vi "Insert Channels and Preserve Value.vi"(7 "channel block":T1 {"buffer offset" format="%d bytes"}, 8 "error in (no error)":errorcluster, 9 "channels buffer index in":u64, 10 "channels buffer in":dbl[](array[numeric]), 11 "Buffer in":refnum<class "Memory Buffer.lvclass">) -> (0 "error out":errorcluster, 1 "channels buffer index out":u64, 2 "channels buffer out":dbl[](array[numeric]), 3 "Buffer out":refnum<class "Memory Buffer.lvclass">)   [LabVIEW 2017, in "Data Sharing Framework Engine.lvlib" / "Memory Buffer.lvclass"]
uses:
  Memory Buffer.lvclass
  Type Definitions/DSF Runtime Channel Block.ctl
  Configuration/1.0.0/Public/Controls/DSF Data Type.ctl
  Write 1D Array of U64.vi
  Write 1D Array of U32.vi
  Write 1D Array of U16.vi
  Write 1D Array of U8.vi
  Write 1D Array of I64.vi
  Write 1D Array of I32.vi
  Write 1D Array of I16.vi
  Write 1D Array of I8.vi
  Write 1D Array of Double.vi
  Write 1D Array of Single.vi
  Write 1D Array of Boolean.vi
  Data Sharing Framework Engine.lvlib
  Configuration/1.0.0/Data Sharing Framework Configuration.lvlib
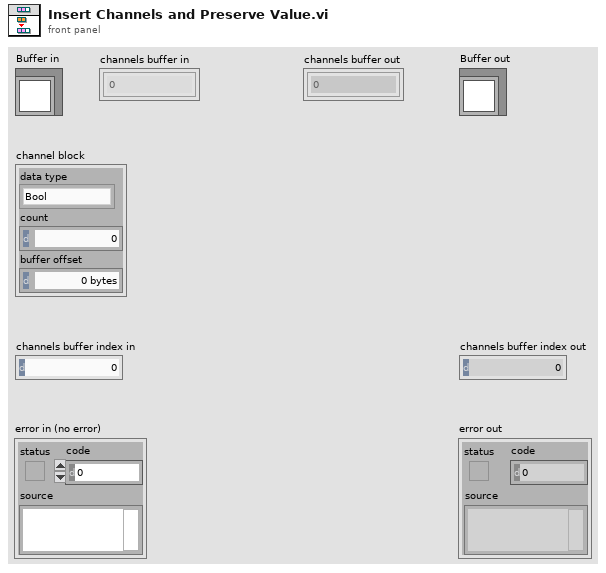
[diagram p1: front panel]
types:
  T1 = typedef "Data Sharing Framework Engine.lvlib/DSF Runtime Channel Block.ctl" = cluster{"data type":T2, "count":u64, "buffer offset":u64}
  T2 = typedef "Data Sharing Framework Configuration.lvlib/DSF Data Type.ctl" = enum8{"Bool", "SGL", "DBL", "I8", "I16", "I32", "I64", "U8", "U16", "U32", "U64"}
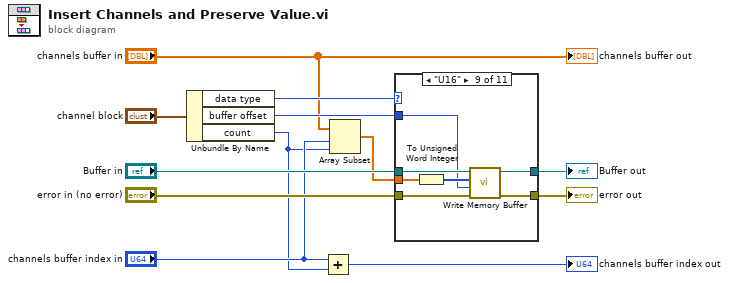
[diagram p0: block diagram]
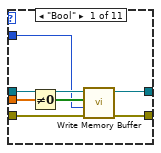
[diagram p2: hidden frame]
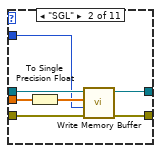
[diagram p3: hidden frame]
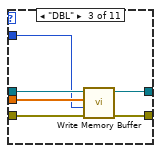
[diagram p4: hidden frame]
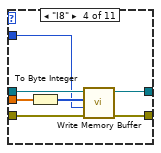
[diagram p5: hidden frame]
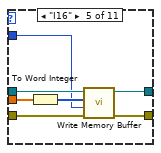
[diagram p6: hidden frame]
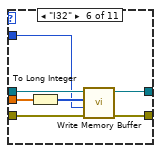
[diagram p7: hidden frame]
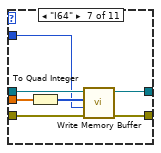
[diagram p8: hidden frame]
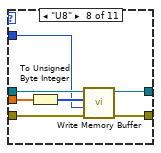
[diagram p9: hidden frame]
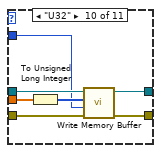
[diagram p10: hidden frame]
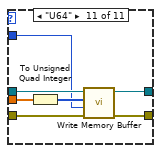
[diagram p11: hidden frame]
diagram:
  n1 = Unbundle By Name("channel block") -> ("data type"=w9:T2, "buffer offset"=w12:u64, "count"=w2:u64)
  n2 = Add(x="channels buffer index in", y=w2) -> (x+y=→"channels buffer index out":u64)
  n3 = Array Subset(array="channels buffer in", index="channels buffer index in", length=w2) -> (w6:dbl[])
  n4 = case shown="\"U16\"" w9 {
    tunnel: "Buffer in" -> [w19 w26 w32 w39 w46 w53 w60 w67 w74 w81 w88]
    tunnel: w6 -> [w14 w21 w28 w34 w41 w48 w55 w62 w69 w76 w83]
    tunnel: "error in (no error)" -> [w18 w25 w31 w38 w45 w52 w59 w66 w73 w80 w87]
    tunnel: [w17 w24 w30 w37 w44 w51 w58 w65 w72 w79 w86] -> w10
    tunnel: w12 -> [w15 w22 w27 w35 w42 w49 w56 w63 w70 w77 w84]
    tunnel: [w13 w20 w29 w33 w40 w47 w54 w61 w68 w75 w82] -> w7
    frame "Bool" {
      n5 = Not Equal To 0?(x=w14) -> (x != 0?=w16:bool[])
      n6 = call-poly "Write Memory Buffer.vi"("error in (no error)"=w18, "offset (0)"=w15, "buffer in"=w16, "Buffer in"=w19) -> ("error out"=w17:errorcluster, "Buffer out"=w13:refnum<class "Memory Buffer.lvclass">)  [unwired: 4 in, 2 out]
    }
    frame "SGL" {
      n7 = To Single Precision Float(number=w21) -> (single precision float=w23:sgl[])
      n8 = call-poly "Write Memory Buffer.vi"("error in (no error)"=w25, "offset (0)"=w22, "buffer in"=w23, "Buffer in"=w26) -> ("error out"=w24:errorcluster, "Buffer out"=w20:refnum<class "Memory Buffer.lvclass">)  [unwired: 4 in, 2 out]
    }
    frame "DBL" {
      n9 = call-poly "Write Memory Buffer.vi"("error in (no error)"=w31, "offset (0)"=w27, "buffer in"=w28, "Buffer in"=w32) -> ("error out"=w30:errorcluster, "Buffer out"=w29:refnum<class "Memory Buffer.lvclass">)  [unwired: 4 in, 2 out]
    }
    frame "I8" {
      n10 = To Byte Integer(number=w34) -> (8bit integer=w36:i8[])
      n11 = call-poly "Write Memory Buffer.vi"("error in (no error)"=w38, "offset (0)"=w35, "buffer in"=w36, "Buffer in"=w39) -> ("error out"=w37:errorcluster, "Buffer out"=w33:refnum<class "Memory Buffer.lvclass">)  [unwired: 4 in, 2 out]
    }
    frame "I16" {
      n12 = To Word Integer(number=w41) -> (16bit integer=w43:i16[])
      n13 = call-poly "Write Memory Buffer.vi"("error in (no error)"=w45, "offset (0)"=w42, "buffer in"=w43, "Buffer in"=w46) -> ("error out"=w44:errorcluster, "Buffer out"=w40:refnum<class "Memory Buffer.lvclass">)  [unwired: 4 in, 2 out]
    }
    frame "I32" {
      n14 = To Long Integer(number=w48) -> (32bit integer=w50:i32[])
      n15 = call-poly "Write Memory Buffer.vi"("error in (no error)"=w52, "offset (0)"=w49, "buffer in"=w50, "Buffer in"=w53) -> ("error out"=w51:errorcluster, "Buffer out"=w47:refnum<class "Memory Buffer.lvclass">)  [unwired: 4 in, 2 out]
    }
    frame "I64" {
      n16 = To Quad Integer(1:w55) -> (0:w57:i64[])
      n17 = call-poly "Write Memory Buffer.vi"("error in (no error)"=w59, "offset (0)"=w56, "buffer in"=w57, "Buffer in"=w60) -> ("error out"=w58:errorcluster, "Buffer out"=w54:refnum<class "Memory Buffer.lvclass">)  [unwired: 4 in, 2 out]
    }
    frame "U8" {
      n18 = To Unsigned Byte Integer(number=w62) -> (unsigned 8bit integer=w64:u8[])
      n19 = call-poly "Write Memory Buffer.vi"("error in (no error)"=w66, "offset (0)"=w63, "buffer in"=w64, "Buffer in"=w67) -> ("error out"=w65:errorcluster, "Buffer out"=w61:refnum<class "Memory Buffer.lvclass">)  [unwired: 4 in, 2 out]
    }
    frame "U16" {
      n20 = To Unsigned Word Integer(number=w69) -> (unsigned 16bit integer=w71:u16[])
      n21 = call-poly "Write Memory Buffer.vi"("error in (no error)"=w73, "offset (0)"=w70, "buffer in"=w71, "Buffer in"=w74) -> ("error out"=w72:errorcluster, "Buffer out"=w68:refnum<class "Memory Buffer.lvclass">)  [unwired: 4 in, 2 out]
    }
    frame "U32" {
      n22 = To Unsigned Long Integer(number=w76) -> (unsigned 32bit integer=w78:u32[])
      n23 = call-poly "Write Memory Buffer.vi"("error in (no error)"=w80, "offset (0)"=w77, "buffer in"=w78, "Buffer in"=w81) -> ("error out"=w79:errorcluster, "Buffer out"=w75:refnum<class "Memory Buffer.lvclass">)  [unwired: 4 in, 2 out]
    }
    frame "U64" {
      n24 = To Unsigned Quad Integer(1:w83) -> (0:w85:u64[])
      n25 = call-poly "Write Memory Buffer.vi"("error in (no error)"=w87, "offset (0)"=w84, "buffer in"=w85, "Buffer in"=w88) -> ("error out"=w86:errorcluster, "Buffer out"=w82:refnum<class "Memory Buffer.lvclass">)  [unwired: 4 in, 2 out]
    }
  }
  "error out" <- w10
  "Buffer out" <- w7
  "channels buffer out" <- "channels buffer in"
